vi "GET_send_ServoStatus_toClient.vi"(3 "LabVIEW Web Service Request":refnum<class "Web Request.lvclass">) -> (2 "status":cluster{"mode":string, "position":dbl})   [LabVIEW 2024]
uses:
  <vilib>/wsapi/Web Request.lvclass
  DataTypes/OperationTypeForFunctionalGlobalVariable.ctl
panel:
  # "Use the Web Service Request input terminal to call the VIs on the Web Services palette. Do not remove it from the connector pane unless you don't need access to the palette."
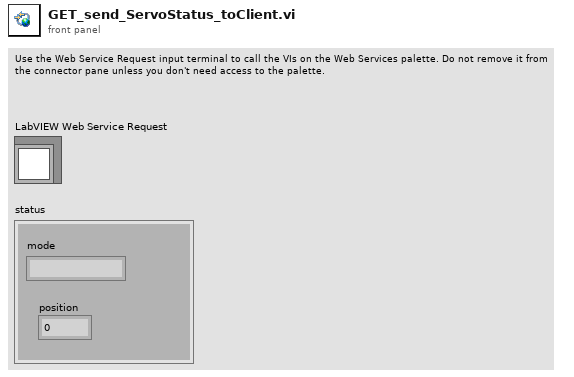
[diagram p1: front panel]
types:
  T1 = typedef "OperationTypeForFunctionalGlobalVariable.ctl" = enum16{"GET", "SET"}
  T2 = typedef "ServoStatus.ctl" = cluster{"mode":string, "position":i16}
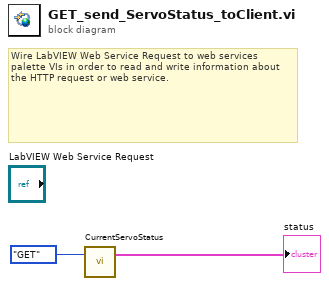
[diagram p0: block diagram]
diagram:
  # "Wire LabVIEW Web Service Request to web services palette VIs in order to read and write information about the HTTP request or web service."
  n1 = call "CurrentServoStatus.vi"("Operation"=OperationTypeForFunctionalGlobalVariable."GET") -> ("Current Servo Status"=→"status":T2)  [unwired: 2 in]
